vi "createdAt.get.vi"(8 "error in (no error)":errorcluster, 11 "Run in":refnum<class "Run.lvclass">) -> (0 "error out":errorcluster, 2 "createdAt":timestamp format="%<%x %.3X>T", 3 "Run out":refnum<class "Run.lvclass">)   [LabVIEW 2020, in "Run.lvclass"]
uses:
  Run.lvclass
  Run.lvclass/Run.ctl
  <vilib>/LabVIEW Open Source Project/Epoch Date & Time/formatter.iso8601/ISO8601 DateString to Timestamp.vi
  Nominal Client/Nominal Client.lvclass
  b3b51881-3115-4bdb-b91c-b9f37aeec093.vi
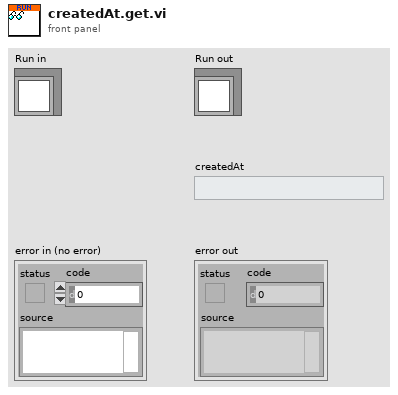
[diagram p1: front panel]
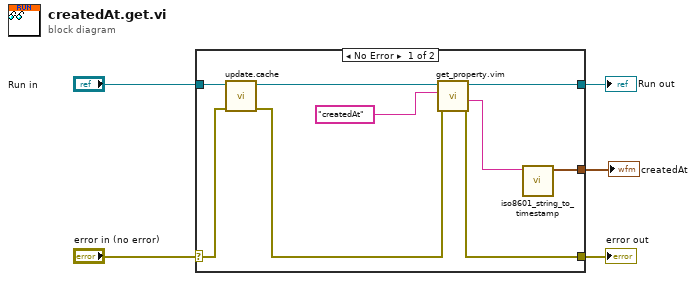
[diagram p0: block diagram]
diagram:
  n1 = case shown="No Error" "error in (no error)" {
    selector: "error in (no error)" -> [w14 w15]
    tunnel: [w6 w15] -> w4
    tunnel: [w8 w16] -> w2
    tunnel: "Run in" -> [w12 w16]
    tunnel: [w13 _] -> w1
    frame No Error {
      n2 = call "update.cache.vi"("error in"=w14, "Run in"=w12) -> ("error out"=w7:errorcluster, "Run out"=w9:refnum<class "Run.lvclass">)  [unwired: 8 in]
      n3 = call "get_property.vim"("error in"=w7, "Property Name"="createdAt", "Run in"=w9) -> ("error out"=w6:errorcluster, "Value"=w10:string, "Run out"=w8:refnum<class "Run.lvclass">)  [unwired: 6 in]
      n4 = call "iso8601_string_to_timestamp.vi"("ISO8601 Timestamp String"=w10) -> ("Time Stamp"=w13:timestamp)  [unwired: 9 in, 1 out]
    }
    frame Error {
    }
  }
  "error out" <- w4
  "Run out" <- w2
  "createdAt" <- w1
